vi "CVT2GroupReadTest.vi"() -> (3 "Unit Test Framework Results":T1)   [LabVIEW 2013, in "UnitTests.lvlib"]
uses:
  UnitTests.lvlib
  <vilib>/utf/common/utf_test_result_troll.ctl
  <vilib>/utf/common/utf_test_result.ctl
  <vilib>/utf/common/utf_test_result_failure.ctl
  <vilib>/utf/common/utf_test_comparison_operators.ctl
  <vilib>/utf/common/utf_vi_tag.ctl
  <vilib>/NI/Current Value Table/Read tags into grouped data.vi
  <vilib>/NI/Current Value Table/Read Index Set.vi
  <vilib>/NI/Current Value Table/DataTypes/Double_Read Index Set.vi
  <vilib>/NI/Current Value Table/DataTypes/Array of String_Read Index Set.vi
  <vilib>/NI/Current Value Table/DataTypes/Array of Boolean_Read Index Set.vi
  <vilib>/NI/Current Value Table/DataTypes/Array of Single_Read Index Set.vi
  <vilib>/NI/Current Value Table/DataTypes/Array of Double_Read Index Set.vi
  <vilib>/NI/Current Value Table/DataTypes/Array of I8_Read Index Set.vi
  <vilib>/NI/Current Value Table/DataTypes/Array of I16_Read Index Set.vi
  <vilib>/NI/Current Value Table/DataTypes/Array of I32_Read Index Set.vi
  <vilib>/NI/Current Value Table/DataTypes/Array of I64_Read Index Set.vi
  <vilib>/NI/Current Value Table/DataTypes/Array of U64_Read Index Set.vi
  <vilib>/NI/Current Value Table/DataTypes/Array of U32_Read Index Set.vi
  <vilib>/NI/Current Value Table/DataTypes/Array of U16_Read Index Set.vi
  <vilib>/NI/Current Value Table/DataTypes/Array of U8_Read Index Set.vi
  <vilib>/NI/Current Value Table/DataTypes/Boolean_Read Index Set.vi
  <vilib>/NI/Current Value Table/DataTypes/String_Read Index Set.vi
  <vilib>/NI/Current Value Table/DataTypes/U8_Read Index Set.vi
  <vilib>/NI/Current Value Table/DataTypes/U16_Read Index Set.vi
  <vilib>/NI/Current Value Table/DataTypes/U32_Read Index Set.vi
  <vilib>/NI/Current Value Table/DataTypes/U64_Read Index Set.vi
  <vilib>/NI/Current Value Table/DataTypes/I8_Read Index Set.vi
  <vilib>/NI/Current Value Table/DataTypes/I16_Read Index Set.vi
  <vilib>/NI/Current Value Table/DataTypes/I32_Read Index Set.vi
  <vilib>/NI/Current Value Table/DataTypes/I64_Read Index Set.vi
  <vilib>/NI/Current Value Table/DataTypes/Single_Read Index Set.vi
  <vilib>/NI/Current Value Table/FGVs/Group Memory.vi
  <vilib>/NI/Current Value Table/Memory Block.vi
  <vilib>/NI/Current Value Table/DataTypes/Double_Memory Block.vi
  <vilib>/NI/Current Value Table/DataTypes/Array of String_Memory Block.vi
  <vilib>/NI/Current Value Table/DataTypes/Array of Boolean_Memory Block.vi
  <vilib>/NI/Current Value Table/DataTypes/Array of Single_Memory Block.vi
  <vilib>/NI/Current Value Table/DataTypes/Array of Double_Memory Block.vi
  <vilib>/NI/Current Value Table/DataTypes/Array of I8_Memory Block.vi
  <vilib>/NI/Current Value Table/DataTypes/Array of I16_Memory Block.vi
  <vilib>/NI/Current Value Table/DataTypes/Array of I32_Memory Block.vi
  <vilib>/NI/Current Value Table/DataTypes/Array of I64_Memory Block.vi
  <vilib>/NI/Current Value Table/DataTypes/Array of U64_Memory Block.vi
  <vilib>/NI/Current Value Table/DataTypes/Array of U32_Memory Block.vi
  <vilib>/NI/Current Value Table/DataTypes/Array of U16_Memory Block.vi
  <vilib>/NI/Current Value Table/DataTypes/Array of U8_Memory Block.vi
  <vilib>/NI/Current Value Table/DataTypes/Boolean_Memory Block.vi
  <vilib>/NI/Current Value Table/DataTypes/String_Memory Block.vi
  <vilib>/NI/Current Value Table/DataTypes/U8_Memory Block.vi
  <vilib>/NI/Current Value Table/DataTypes/U16_Memory Block.vi
  <vilib>/NI/Current Value Table/DataTypes/U32_Memory Block.vi
  <vilib>/NI/Current Value Table/DataTypes/U64_Memory Block.vi
  <vilib>/NI/Current Value Table/DataTypes/I8_Memory Block.vi
  <vilib>/NI/Current Value Table/DataTypes/I16_Memory Block.vi
  <vilib>/NI/Current Value Table/DataTypes/I32_Memory Block.vi
  <vilib>/NI/Current Value Table/DataTypes/I64_Memory Block.vi
  <vilib>/NI/Current Value Table/DataTypes/Single_Memory Block.vi
  <vilib>/utf/NI_UnitTestFramework.lvlib
  <vilib>/NI/Current Value Table/Current Value Table.lvlib
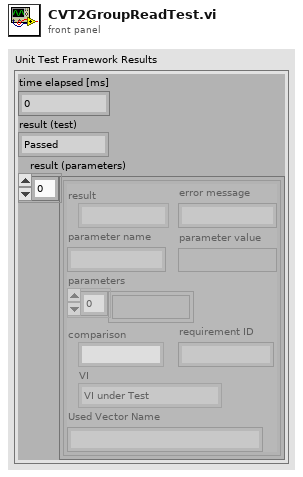
[diagram p1: front panel]
types:
  T1 = typedef "NI_UnitTestFramework.lvlib/utf_test_result_troll.ctl" = cluster{"time elapsed [ms]":u32, "result (test)":T2, "result (parameters)":T3[]}
  T2 = typedef "NI_UnitTestFramework.lvlib/utf_test_result.ctl" = enum16{"Passed", "Failed", "Error", "Skipped", "Not Processed"}
  T3 = typedef "NI_UnitTestFramework.lvlib/utf_test_result_failure.ctl" = cluster{"result":T2, "error message":string, "parameter name":string, "parameter value":variant, "parameters":variant[], "comparison":T4, "requirement ID":string, "VI":T5, "Used Vector Name":string}
  T4 = typedef "NI_UnitTestFramework.lvlib/utf_test_comparison_operators.ctl" = enum16{"=", "!=", ">", ">=", "<", "<=", "range", "symmetric tolerance", "asymmetric tolerance", "string contains", "string not contain", "array size", "string length", "array range", "by element", "array range (limit array)", "user-defined", "array contains", "array not contain", "vector length", "= (elm)", "!= (elm)", "= (case insensitive)", "!= (case insensitive)"}
  T5 = typedef "NI_UnitTestFramework.lvlib/utf_vi_tag.ctl" = enum16{"Setup VI", "VI under Test", "Teardown VI"}
  T6 = typedef "Current Value Table.lvlib/Group Data.ctl" = cluster{"Double":dbl[], "Single":sgl[], "I64":i64[], "I32":i32[], "I16":i16[], "I8":i8[], "U64":u64[], "U32":u32[], "U16":u16[], "U8":u8[], "String":string[], "Boolean":bool[], "Array of U8":cluster{"U8 Array":u8[]}[], "Array of U16":cluster{"U16 Array":u16[]}[], "Array of U32":cluster{"U32 Array":u32[]}[], "Array of U64":cluster{"U64 Array":u64[]}[], "Array of I64":cluster{"I64 Array":i64[]}[], "Array of I32":cluster{"I32 Array":i32[]}[], "Array of I16":cluster{"I16 Array":i16[]}[], "Array of I8":cluster{"I8 Array":i8[]}[], "Array of Double":cluster{"DBL Array":dbl[]}[], "Array of Single":cluster{"SGL Array":sgl[]}[], "Array of Boolean":cluster{"Boolean Array":bool[]}[], "Array of String":cluster{"String Array":string[]}[]}
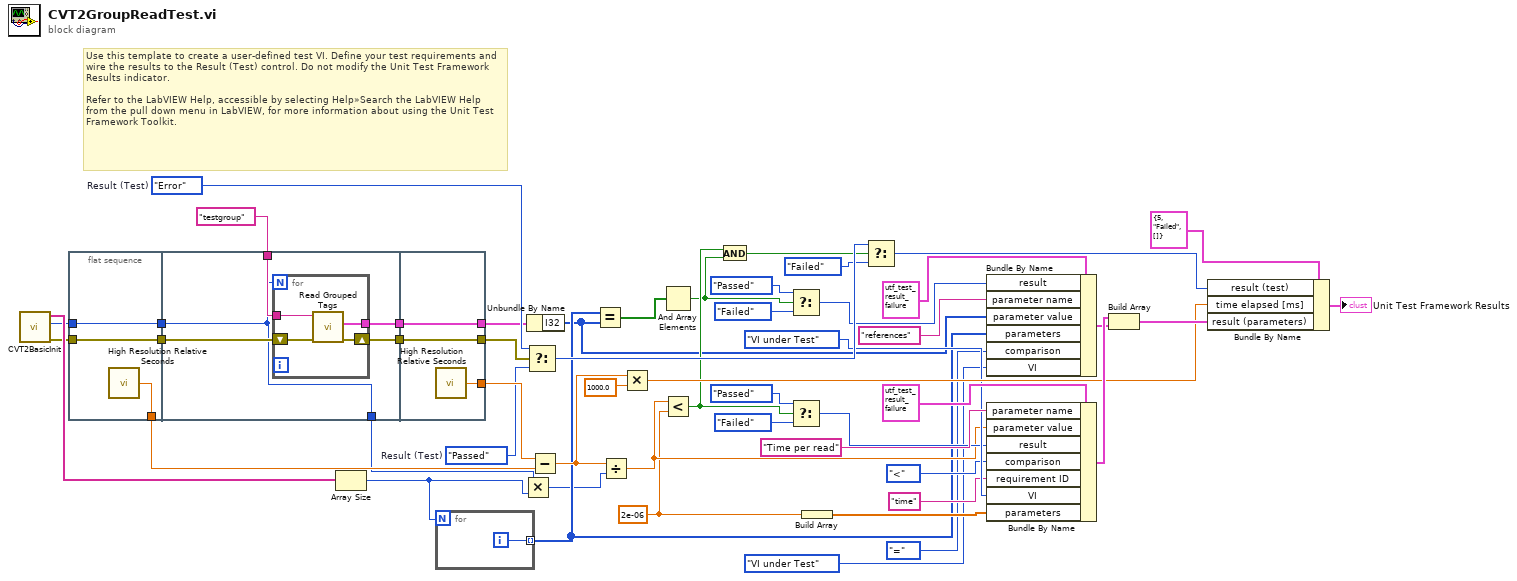
[diagram p0: block diagram]
diagram:
  w26 = 2e-06 ("y")
  w47 = utf_test_result."Error"  # Result (Test)
  w46 = utf_test_result."Passed"  # Result (Test)
  # "Use this template to create a user-defined test VI. Define your test requirements and wire the results to the Result (Test) control. Do not modify the Unit Test Framework Results indicator. \n\nRefer to the LabVIEW Help, accessible by selecting Help»Search the LabVIEW Help from the pull down menu in LabVIEW, for more information about using the Unit Test Framework Toolkit."
  n1 = call "CVT2BasicInit.vi"() -> ("error out"=w8:errorcluster, "Tags per type out"=w4:i32, "names"=w20:string[])  [unwired: 9 in]
  n2 = flat-sequence {
    tunnel: [w55] -> w49
    tunnel: w8 -> [w53]
    tunnel: [w54] -> w41
    tunnel: w4 -> [w54]
    tunnel: [w53] -> w40
    tunnel: w41 -> [w56]
    tunnel: w40 -> [w60]
    tunnel: [w59] -> w39
    tunnel: [w58] -> w21
    tunnel: "testgroup" ("Group") -> [w57]
    tunnel: [w56] -> w1
    tunnel: [w67] -> w50
    tunnel: w39 -> [w66]
    tunnel: [w66] -> w7
    tunnel: [w65] -> w6
    tunnel: w21 -> [w65]
    frame #0 {
      n3 = call <vilib>:"High Resolution Relative Seconds.vi"() -> ("relative seconds"=w55:dbl)
    }
    frame #1 {
      n4 = for {
        N: w56 -> [_]
        shift-right: [w63] -> w59
        shift-left: w60 -> [w64]
        tunnel: [w62] -> w58
        tunnel: w57 -> [w61]
        n5 = call <vilib>:"Read Grouped Tags.vi"("error in (no error)"=w64, "Group"=w61) -> ("error out"=w63:errorcluster, "Data"=w62:T6)  [unwired: 8 in]
      }
    }
    frame #2 {
      n6 = call <vilib>:"High Resolution Relative Seconds.vi"() -> ("relative seconds"=w67:dbl)
    }
  }
  n7 = Array Size(array=w20) -> (size(s)=w2:i32)
  n8 = for {
    N: w2 -> [_]
    tunnel: [w68] -> w10 mode=indexing
    i -> [w68]
  }
  n9 = Multiply(x=w1, y=w2) -> (x*y=w3:i32)
  n10 = Unbundle By Name(w6) -> ("I32"=w5:i32[])
  n11 = Select(t=w47, s=w7, f=w46) -> (s? t:f=w36:T2)
  n12 = Subtract(x=w50, y=w49) -> (x-y=w38:dbl)
  n13 = Equal?(x=w10, y=w5) -> (x = y?=w12:bool[])
  n14 = Divide(x=w38, y=w3) -> (x/y=w29:dbl)
  n15 = Multiply(x=w38, y=1000.0) -> (x*y=w42:dbl)
  n16 = And Array Elements(Boolean array=w12) -> (logical AND=w11:bool)
  n17 = Less?(x=w29, y=w26) -> (x < y?=w22:bool)
  n18 = And(x=w22, y=w11) -> (x .and. y?=w23:bool)
  n19 = Select(t=utf_test_result."Passed" ("result"), s=w11, f=utf_test_result."Failed" ("result")) -> (s? t:f=w15:T2)
  n20 = Select(t=utf_test_result."Passed" ("result"), s=w22, f=utf_test_result."Failed" ("result")) -> (s? t:f=w30:T2)
  n21 = Build Array(w26) -> (w25:dbl[])
  n22 = Select(t=w36, s=w23, f=utf_test_result."Failed") -> (s? t:f=w34:T2)
  n23 = Bundle By Name(cluster=T3 {"result"=enum."Passed", "error message"="", "parameter name"="", "parameter value"=variant, "parameters"=[], "comparison"=enum."=", "requirement ID"="", "VI"=enum."Setup VI", "Used Vector Name"=""} ("Unit Test Framework - result (parameters)"), "result"=w15, "parameter name"="references" ("format string"), "parameter value"=w5, "parameters"=w10, "comparison"=utf_test_comparison_operators."=", "VI"=utf_vi_tag."VI under Test") -> (w24:T3)
  n24 = Bundle By Name(cluster=T3 {"result"=enum."Passed", "error message"="", "parameter name"="", "parameter value"=variant, "parameters"=[], "comparison"=enum."=", "requirement ID"="", "VI"=enum."Setup VI", "Used Vector Name"=""} ("Unit Test Framework - result (parameters)"), "parameter name"="Time per read", "parameter value"=w29, "result"=w30, "comparison"=utf_test_comparison_operators."<", "requirement ID"="time", "VI"=utf_vi_tag."VI under Test", "parameters"=w25) -> (w45:T3)
  n25 = Build Array(w45, w24) -> (w44:T3[])
  n26 = Bundle By Name(cluster=T1 {"time elapsed [ms]"=5, "result (test)"=enum."Failed", "result (parameters)"=[]} ("Unit Test Framework - Result"), "result (test)"=w34, "time elapsed [ms]"=w42, "result (parameters)"=w44) -> (→"Unit Test Framework Results":T1)
